vi "Generate Command Parameters.vi"(7 "Instrument Addon Refnum in":T1 format="%.0x", 8 "Error In":errorcluster, 10 "Command String":string, 11 "Command Channel in":T1 format="%.0x") -> (0 "Error Out":errorcluster, 1 "Wait Channel Ref out":T1 format="%.0x", 2 "Linked Channels":T2[](array[typedef]) {"Channel Refnum" format="%.0x"}, 3 "Command Channel out":T1 format="%.0x")   [LabVIEW 2018, in "Instrument Addon Scripting API Messages Unit Tests.lvclass"]
uses:
  Instrument Addon Scripting API Messages Unit Tests.lvclass
  <vilib>/NI Veristand/Custom Device API/Custom Device Item Ref.ctl
  APIs/Scripting API/TypeDefs/Linked Channel.ctl
  Addon/Addon Shared/SubVIs/Constants.vi
  <vilib>/NI/NI VeriStand Advanced SysDef API/_SubVIs/SysDef.Search.GUID.vi
  <vilib>/NI Veristand/Custom Device API/Custom Device API.lvlib
  APIs/Scripting API/Instrument Addon Scripting API.lvlib
  <vilib>/NI/NI VeriStand Advanced SysDef API/SysDef API/Advanced System Definition.lvlib
  Addon/Addon Shared/Instrument Addon Shared.lvlib
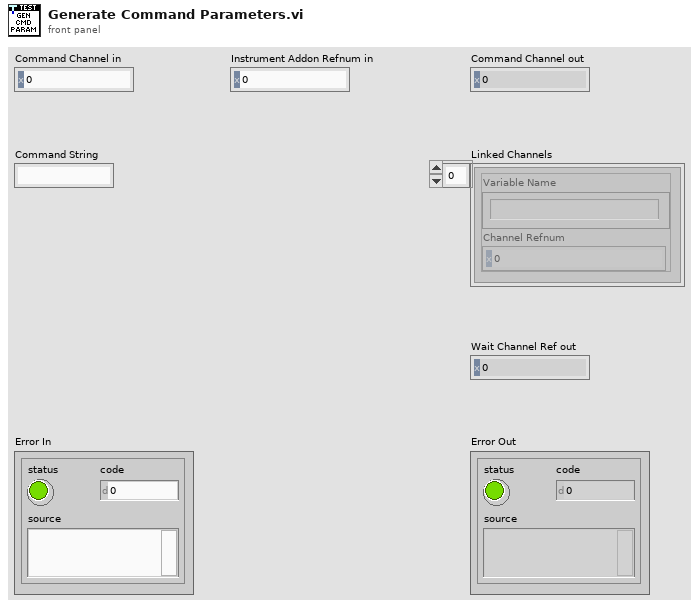
[diagram p1: front panel]
types:
  T1 = typedef "Custom Device API.lvlib/Custom Device Item Ref.ctl" = u64
  T2 = typedef "Instrument Addon Scripting API.lvlib/Linked Channel.ctl" = cluster{"Variable Name":string, "Channel Refnum":T1}
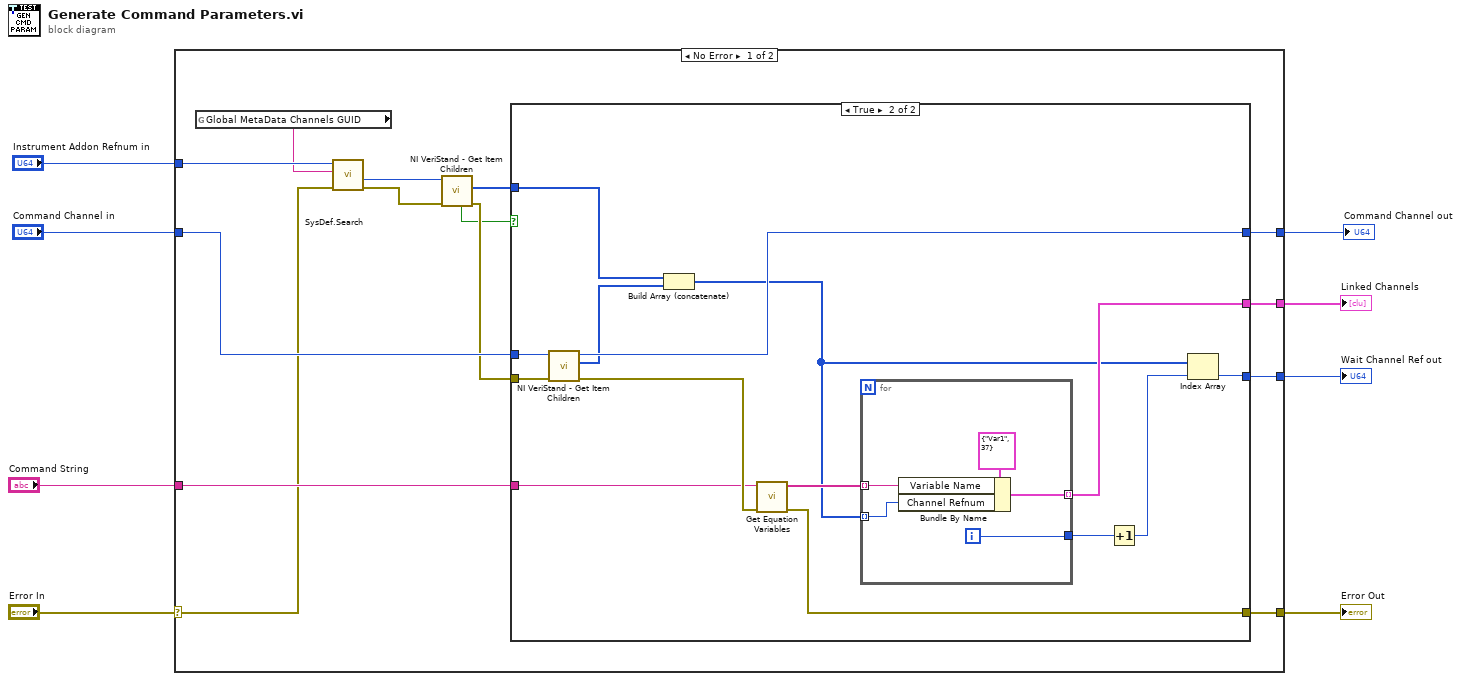
[diagram p0: block diagram]
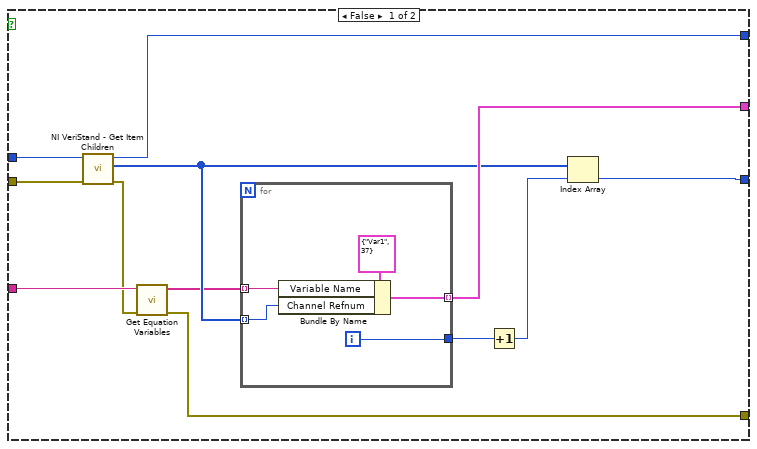
[diagram p2: hidden frame]
diagram:
  n1 = case shown="No Error" "Error In" {
    selector: "Error In" -> [w11 w60]
    tunnel: [w22 _] -> w8
    tunnel: [w21 _] -> w7
    tunnel: "Command String" -> [w18 _]
    tunnel: [w17 w60] -> w4
    tunnel: "Command Channel in" -> [w20 w59]
    tunnel: [w19 w59] -> w2
    tunnel: "Instrument Addon Refnum in" -> [w13 _]
    frame No Error {
      n2 = global read "Constants.vi" "Global MetaData Channels GUID"() -> (w9:string)
      n3 = call-poly <vilib>:"SysDef.Search.vi"("error in (no error)"=w11, "GUID"=w9, "nodeID"=w13) -> ("error out"=w10:errorcluster, "Value out"=w12:u64)  [unwired: 5 in, 2 out]
      n4 = call <vilib>:"NI VeriStand - Get Item Children.vi"("error in (no error)"=w10, "Item Ref in"=w12) -> ("error out"=w16:errorcluster, "Child Refs"=w14:T1[], "Found"=w15:bool)  [unwired: 6 in, 1 out]
      n5 = case shown="True" w15 {
        tunnel: [w34 w49] -> w22
        tunnel: [w33 w48] -> w21
        tunnel: w20 -> [w30 w44]
        tunnel: [w28 w47] -> w19
        tunnel: w18 -> [w27 w45]
        tunnel: [w24 w46] -> w17
        tunnel: w16 -> [w23 w43]
        tunnel: w14 -> [_ w42]
        frame False {
          n6 = call <vilib>:"NI VeriStand - Get Item Children.vi"("error in (no error)"=w23, "Item Ref in"=w30) -> ("error out"=w25:errorcluster, "Child Refs"=w29:T1[], "Item Ref out"=w28:T1)  [unwired: 6 in, 1 out]
          n7 = call "Get Equation Variables.vi"("error in (no error)"=w25, "Format String"=w27) -> ("error out"=w24:errorcluster, "Variables out"=w26:string[])  [unwired: 7 in, 1 out]
          n8 = for {
            tunnel: w26 -> [w38] mode=indexing
            tunnel: w29 -> [w37] mode=indexing
            tunnel: [w36] -> w33 mode=indexing
            tunnel: [w35] -> w31
            i -> [w35]
            n9 = Bundle By Name(cluster=T2 {"Variable Name"="Var1", "Channel Refnum"=37} ("Linked Channel"), "Variable Name"=w38, "Channel Refnum"=w37) -> (w36:T2)
          }
          n10 = Increment(x=w31) -> (x+1=w32:i32)
          n11 = Index Array(array=w29, index=w32) -> (element=w34:T1)
        }
        frame True {
          n12 = call <vilib>:"NI VeriStand - Get Item Children.vi"("error in (no error)"=w43, "Item Ref in"=w44) -> ("error out"=w50:errorcluster, "Child Refs"=w41:T1[], "Item Ref out"=w47:T1)  [unwired: 6 in, 1 out]
          n13 = Build Array (concatenate)(w42, w41) -> (w40:T1[])
          n14 = call "Get Equation Variables.vi"("error in (no error)"=w50, "Format String"=w45) -> ("error out"=w46:errorcluster, "Variables out"=w51:string[])  [unwired: 7 in, 1 out]
          n15 = for {
            tunnel: w51 -> [w57] mode=indexing
            tunnel: w40 -> [w56] mode=indexing
            tunnel: [w55] -> w48 mode=indexing
            tunnel: [w54] -> w52
            i -> [w54]
            n16 = Bundle By Name(cluster=T2 {"Variable Name"="Var1", "Channel Refnum"=37} ("Linked Channel"), "Variable Name"=w57, "Channel Refnum"=w56) -> (w55:T2)
          }
          n17 = Increment(x=w52) -> (x+1=w53:i32)
          n18 = Index Array(array=w40, index=w53) -> (element=w49:T1)
        }
      }
    }
    frame Error {
    }
  }
  "Wait Channel Ref out" <- w8
  "Linked Channels" <- w7
  "Error Out" <- w4
  "Command Channel out" <- w2
